vi "runscenario run template.vi"(6 "User Information":T3, 7 "Array":string[](array[string]), 8 "error in (no error)":errorcluster, 9 "POST (empty)":T2, 10 "sxScenarioId (\"\")":string, 11 "Connection Refnum":T4) -> (0 "error out":errorcluster, 3 "dup Connection Refnum":T4)   [LabVIEW 2011]
uses:
  Summitek EXT/ODBC/SQL Controls/Connection Refnum.ctl
  server/database/Users/User Record.ctl
  ITK EXT/utils/keyedarr.llb/Keyed Array.ctl
  server/DIAdem/Datasheet/Datasheet Report Info.ctl
panel:
  out "Datasheet Paths":T1[](array[typedef])
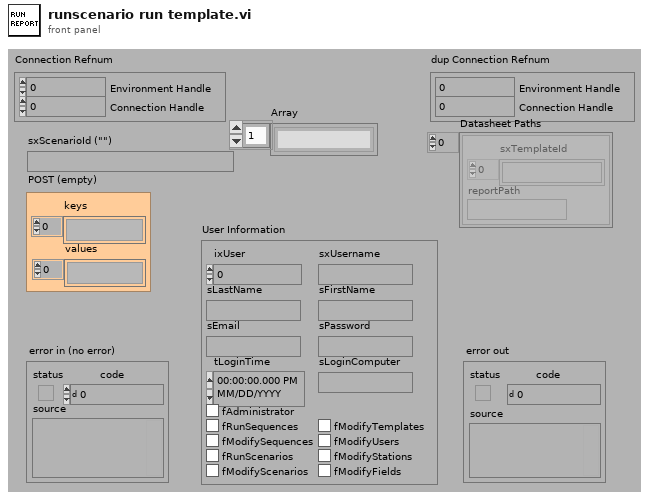
[diagram p1: front panel]
types:
  T1 = typedef "Datasheet Report Info.ctl" = cluster{"sxTemplateId":string[], "reportPath":path}
  T2 = typedef "Keyed Array.ctl" = cluster{"keys":string[], "values":string[]}
  T3 = typedef "User Record.ctl" = cluster{"ixUser":i32, "sxUsername":string, "sLastName":string, "sFirstName":string, "sEmail":string, "sPassword":string, "tLoginTime":timestamp, "sLoginComputer":string, "fAdministrator":bool, "fRunSequences":bool, "fModifySequences":bool, "fRunScenarios":bool, "fModifyScenarios":bool, "fModifyTemplates":bool, "fModifyUsers":bool, "fModifyStations":bool, "fModifyFields":bool}
  T4 = typedef "Connection Refnum.ctl" = cluster{"Environment Handle":i32, "Connection Handle":i32}
  T5 = enum16{"open", "replace", "create", "open or create", "replace or create", "replace or create with confirmation"}
  T6 = typedef "Scenario Record.ctl" = cluster{"ixScenario":i32, "tCreated":timestamp, "tModified":timestamp, "sxUsername":string, "sModifiedBy":string, "sxScenarioId":string, "sDescription":string, "sLogic":string, "sResultFieldsCSV":string, "sTemplatesCSV":string, "fAutoRunReports":bool, "fSortByTemplates":bool, "fCombinePDF":bool, "Conditions":T7[]}
  T7 = typedef "Condition Record.ctl" = cluster{"iConditionIndex":i32, "sxFieldId":string, "nOperator":T8, "sMatchValue":string}
  T8 = typedef "Condition Operators.ctl" = enum16{"equal (=)", "not equal (\\u2260)", "less than (<)", "less than or equal (\\u2264)", "greater than (>)", "greater than or equal (\\u2265)", "contains", "does not contain"}
  T9 = typedef "Template Record.ctl" = cluster{"ixTemplate":i32, "sxTemplateId":string, "sDescription":string, "sCreator":string, "tCreationDate":timestamp, "sModifier":string, "tModifiedDate":timestamp, "sType":string, "sStyle":string, "sFormat":string, "dWidth":dbl, "dHeight":dbl, "sFilename":string, "sScript":string, "sLayout":string, "sEditor":string, "sStyleProcess":string}
  T10 = typedef "DATASHEET Generator Settings.ctl" = cluster{"Wait? (t)":bool, "ClientPrint? (f)":bool, "Client (\"\")":string, "joinPDF":bool, "Sort Method":enum16{"Item", "Template", "No Sort"}, "Export Row (-1=all)":i32, "Preview":bool, "Estimate Time":bool, "username":string, "jobid":string}
  T11 = typedef "TDM_INDEX Record.ctl" = cluster{"Model Number":string, "SN for sort":i32, "Test Type":string, "Test Run":string, "Serial Number":string, "Start Timestamp":timestamp, "Data File":path, "Result Columns":string[]}
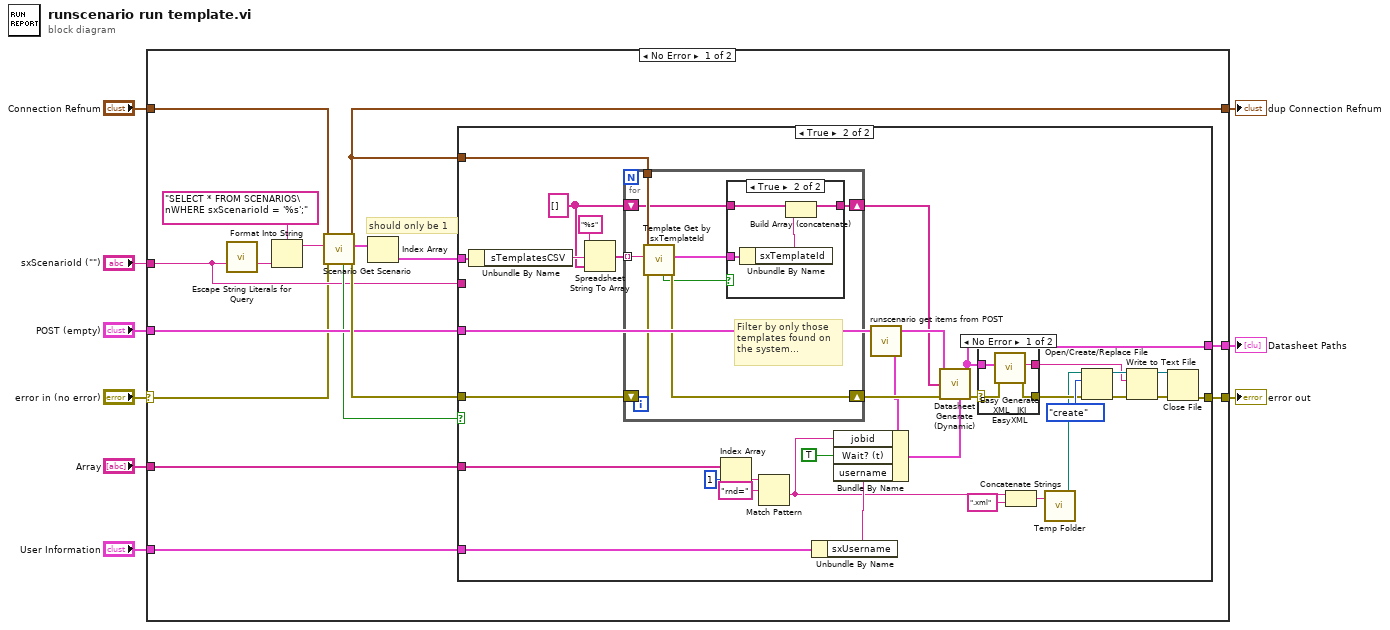
[diagram p0: block diagram]
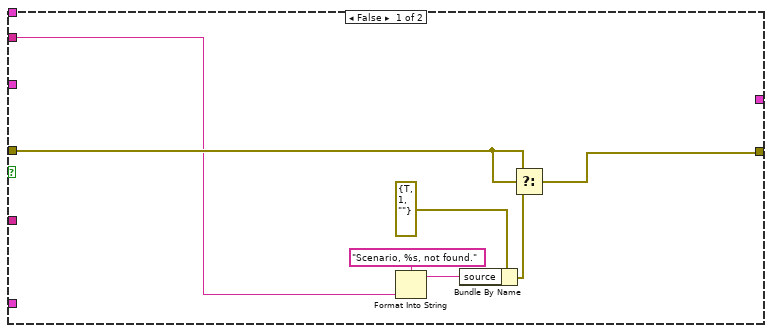
[diagram p2: hidden frame]
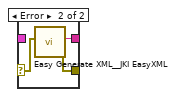
[diagram p3: hidden frame]
diagram:
  n1 = case shown="No Error" "error in (no error)" {
    selector: "error in (no error)" -> [w12 w87]
    tunnel: "Connection Refnum" -> [w25 w88]
    tunnel: [w24 w87] -> w8
    tunnel: "User Information" -> [w23 _]
    tunnel: "POST (empty)" -> [w21 _]
    tunnel: "sxScenarioId (\"\")" -> [w14 _]
    tunnel: [w13 w88] -> w4
    tunnel: "Array" -> [w11 _]
    tunnel: [w10 _] -> w1
    frame No Error {
      # "should only be 1"
      n2 = call "Escape String Literals for Query.vi"("String"=w14) -> ("escaped String"=w18:string)  [unwired: 1 in, 13 out]
      n3 = Format Into String(format string="SELECT * FROM SCENARIOS\nWHERE sxScenarioId = '%s';", w18) -> (resulting string=w17:string)  [unwired: 2 in, 1 out]
      n4 = call "Scenario Get Scenario.vi"("error in (no error)"=w12, "Query"=w17, "Connection Refnum"=w25) -> ("error out"=w22:errorcluster, "Scenarios"=w16:T6[], "Connection Refnum"=w13:T4, "Data Present?"=w20:bool)  [unwired: 5 out]
      n5 = Index Array(array=w16) -> (element=w15:T6)  [unwired: 1 in]
      n6 = case shown="True" w20 {
        tunnel: [w26 w37] -> w24
        tunnel: w23 -> [_ w66]
        tunnel: w22 -> [w32 w58]
        tunnel: w15 -> [_ w65]
        tunnel: w21 -> [_ w63]
        tunnel: w14 -> [w27 _]
        tunnel: w13 -> [_ w60]
        tunnel: w11 -> [_ w40]
        tunnel: [_ w35] -> w10
        frame False {
          n7 = Format Into String(format string="Scenario, %s, not found." ("source"), w27) -> (resulting string=w28:string)  [unwired: 2 in, 1 out]
          n8 = Bundle By Name(cluster=errorcluster {"status"=TRUE, "code"=1, "source"=""} ("error out"), "source"=w28) -> (w29:errorcluster)
          n9 = Select(t=w32, s=w32, f=w29) -> (s? t:f=w26:errorcluster)
        }
        frame True {
          w59 = string[] []
          n10 = Unbundle By Name(w65) -> ("sTemplatesCSV"=w62:string)
          n11 = Spreadsheet String To Array(format string="%s", spreadsheet string=w62, array type (2D Dbl)=w59) -> (array=w52:string[])  [unwired: 1 out]
          n12 = for {
            shift-right: [w78] -> w57
            shift-left: w58 -> [w79]
            tunnel: w52 -> [w81] mode=indexing
            tunnel: w60 -> [w80]
            shift-right: [w74] -> w53
            shift-left: w59 -> [w75]
            # "Filter by only those\ntemplates found on\nthe system..."
            n13 = call "Template Get by sxTemplateId.vi"("error in (no error)"=w79, "sxTemplateId (\"\")"=w81, "Connection Refnum"=w80) -> ("error out"=w78:errorcluster, "Template Record"=w76:T9, "Data Present"=w77:bool)  [unwired: 6 out]
            n14 = case shown="True" w77 {
              tunnel: w76 -> [_ w86]
              tunnel: w75 -> [w82 w85]
              tunnel: [w82 w84] -> w74
              frame False {
              }
              frame True {
                n15 = Unbundle By Name(w86) -> ("sxTemplateId"=w83:string)
                n16 = Build Array (concatenate)(w85, w83) -> (w84:string[])
              }
            }
          }
          n17 = Index Array(array=w40, index=1) -> (element=w43:string)
          n18 = Match Pattern(string=w43, regular expression="rnd=" ("format string")) -> (after substring=w41:string)  [unwired: 1 in, 3 out]
          n19 = Unbundle By Name(w66) -> ("sxUsername"=w54:string)
          n20 = call "runscenario get items from POST.vi"("POST (empty)"=w63) -> ("Generator Settings"=w56:T10, "Items"=w64:T11[])  [unwired: 3 out]
          n21 = Bundle By Name(cluster=w56, "jobid"=w41, "Wait? (t)"=TRUE, "username"=w54) -> (w55:T10)
          n22 = call "Datasheet Generate (Dynamic).vi"("Generator Settings"=w55, "error in (no error)"=w57, "Templates"=w53, "Items"=w64) -> ("error out"=w36:errorcluster, "Datasheet Paths"=w35:T1[])  [unwired: 5 in, 1 out]
          n23 = case shown="No Error" w36 {
            selector: w36 -> [w68 w71]
            tunnel: [w70 w73] -> w39
            tunnel: [w69 w72] -> w38
            tunnel: w35 -> [w67 _]
            frame No Error {
              n24 = call "Easy Generate XML__JKI EasyXML.vi"("error in (no error)"=w68, "LabVIEW Data"=w67) -> ("error out"=w69:errorcluster, "XML String"=w70:string)  [unwired: 8 out]
            }
            frame Error {
              n25 = call "Easy Generate XML__JKI EasyXML.vi"("LabVIEW Data"=w71) -> ("error out"=w72:errorcluster, "XML String"=w73:string)  [unwired: 1 in, 8 out]
            }
          }
          n26 = Concatenate Strings(w41, ".xml" ("string")) -> (w34:string)
          n27 = call "Temp Folder.vi"("Relative Path (\"\")"=w34) -> ("Temp Folder"=w33:path)  [unwired: 2 in]
          n28 = Open/Create/Replace File(file path (use dialog)=w33, error in=w38, operation (0:open)=T5."create") -> (refnum out=w47:refnum<file>, error out=w50:errorcluster)  [unwired: 3 in, 1 out]
          n29 = Write to Text File(file (use dialog)=w47, text=w39, error in=w50) -> (refnum out=w48:refnum<file>, error out=w49:errorcluster)  [unwired: 1 in, 1 out]
          n30 = Close File(refnum=w48, error in=w49) -> (error out=w37:errorcluster)  [unwired: 1 out]
        }
      }
    }
    frame Error {
    }
  }
  "dup Connection Refnum" <- w4
  "error out" <- w8
  "Datasheet Paths" <- w1
